vi "car moving.vi"() -> ()   [LabVIEW 2020]
panel:
  in  "?":bool
  in  "speedometer":dbl(knob)
  out "?":dbl(slide) scale=0.0..1000.0
  # "slow"
  # "speed"
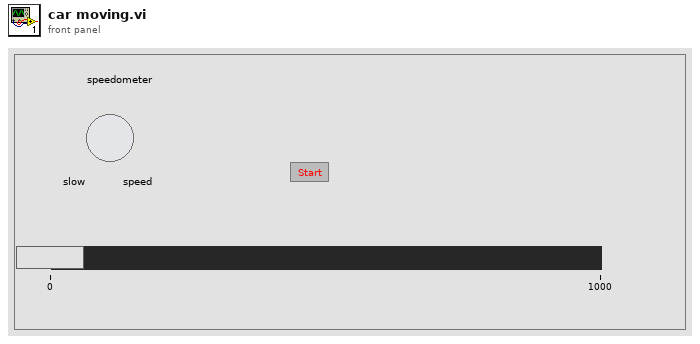
[diagram p1: front panel]
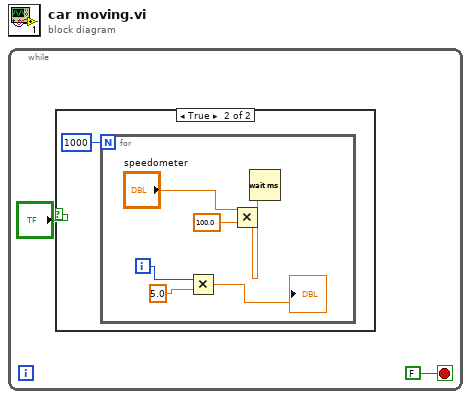
[diagram p0: block diagram]
diagram:
  n1 = while {
    stop <- FALSE stop-if-true
    n2 = case shown="True" "?" {
      frame False {
      }
      frame True {
        n3 = for {
          N: 1000 -> [_]
          i -> [w4]
          n4 = Multiply(x=w4, y=5.0) -> (x*y=→"?":dbl)
          n5 = Multiply(x="speedometer", y=100.0) -> (x*y=w8:dbl)
          n6 = Wait (ms)(milliseconds to wait=w8) -> ()  [unwired: 1 out]
        }
      }
    }
  }
